vi "LKS331GetTemp.vi"(8 "error in (no error)":errorcluster, 11 "LKS Temp Controller":refnum<visa-resource-name>) -> (0 "error out (no error)":errorcluster, 2 "T2":dbl, 3 "T1":dbl)   [LabVIEW 2014]
uses:
  Lake Shore Cryotronics 331/Lake Shore Cryotronics 331.lvlib
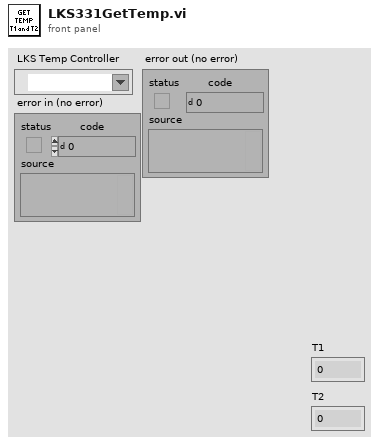
[diagram p1: front panel]
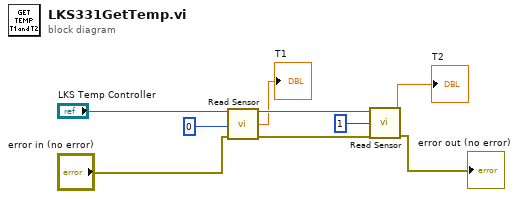
[diagram p0: block diagram]
diagram:
  n1 = call "Read Sensor.vi"("VISA resource name"="LKS Temp Controller", "Input (0: A)"=0, "error in (no error)"="error in (no error)") -> ("VISA resource name out"=w9:refnum<visa-resource-name>, "Kelvin Reading"=→"T1":dbl, "error out"=w7:errorcluster)  [unwired: 8 in, 2 out]
  n2 = call "Read Sensor.vi"("VISA resource name"=w9, "Input (0: A)"=1, "error in (no error)"=w7) -> ("Kelvin Reading"=→"T2":dbl, "error out"=→"error out (no error)":errorcluster)  [unwired: 8 in, 3 out]
